vi "Rec Get Recordset Properties (CR).vi"(4 "error in (no error)":errorcluster, 7 "command-recordset reference":T3) -> (0 "error out":errorcluster, 1 "recordset properties":T1, 3 "command-recordset reference out":T3)   [LabVIEW 2017, in "NI_Database_API.lvlib"]
doc: "Gets properties of the object as determined by the inputs. This VI works for connections, commands, recordsets, columns, and parameters. Wire data to the reference input to determine the polymorphic instance to use or manually select the instance."
uses:
  <vilib>/addons/database/NI_Database_API.lvlib
  <vilib>/addons/database/Command-Recordset.llb/Cmd-Rec Object Reference.ctl
  <vilib>/addons/database/Recordset.llb/Rec Properties.ctl
  <vilib>/addons/database/Auxilliary.llb/DB Tools Cursor Type.ctl
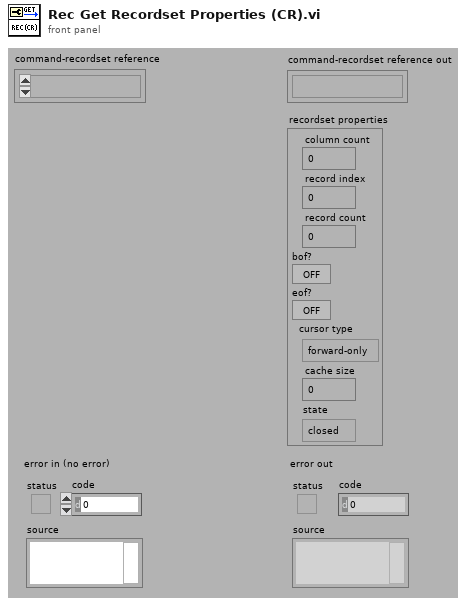
[diagram p1: front panel]
types:
  T1 = typedef "NI_Database_API.lvlib/Rec Properties.ctl" = cluster{"column count":i32, "record index":i32, "record count":i32, "bof?":bool, "eof?":bool, "cursor type":T2, "cache size":i32, "state":enum16{"closed", "open"}}
  T2 = typedef "NI_Database_API.lvlib/DB Tools Cursor Type.ctl" = enum16{"forward-only", "keyset", "dynamic", "static"}
  T3 = typedef "NI_Database_API.lvlib/Cmd-Rec Object Reference.ctl" = refnum<k1>
  T4 = typedef "NI_Database_API.lvlib/Cmd-Rec Data Members.ctl" = cluster{"recordset reference":T5, "command reference":T6}
  T5 = typedef "NI_Database_API.lvlib/Rec ObjectReference.ctl" = refnum<k1>
  T6 = typedef "NI_Database_API.lvlib/Cmd ObjectReference.ctl" = refnum<k1>
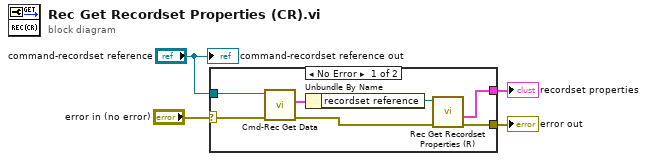
[diagram p0: block diagram]
diagram:
  n1 = case shown="No Error" "error in (no error)" {
    selector: "error in (no error)" -> [w5 w12]
    tunnel: [w11 w12] -> w4
    tunnel: [w10 _] -> w3
    tunnel: "command-recordset reference" -> [w6 _]
    frame No Error {
      n2 = call <vilib>:"Cmd-Rec Get Data.vi"("error in (no error)"=w5, "command-recordset reference"=w6) -> ("error out"=w8:errorcluster, "data"=w7:T4)  [unwired: 2 in, 2 out]
      n3 = Unbundle By Name(w7) -> ("recordset reference"=w9:T5)
      n4 = call <vilib>:"Rec Get Recordset Properties (R).vi"("error in (no error)"=w8, "recordset reference"=w9) -> ("error out"=w11:errorcluster, "recordset properties"=w10:T1)  [unwired: 3 in, 1 out]
    }
    frame Error {
    }
  }
  "error out" <- w4
  "recordset properties" <- w3
  "command-recordset reference out" <- "command-recordset reference"
